vi "Read GUI Events.vi"(8 "error in (no error)":errorcluster, 11 "CS++Scope in":refnum<class "CS++Scope.lvclass">) -> (0 "error out":errorcluster, 2 "GUI Events":cluster{"Stop":refnum<user-event>}, 3 "CS++Scope out":refnum<class "CS++Scope.lvclass">)   [LabVIEW 2016, in "CS++Scope.lvlib" / "CS++Scope.lvclass"]
uses:
  CS++Scope.lvclass
  CS++Scope.lvclass/CS++Scope.ctl
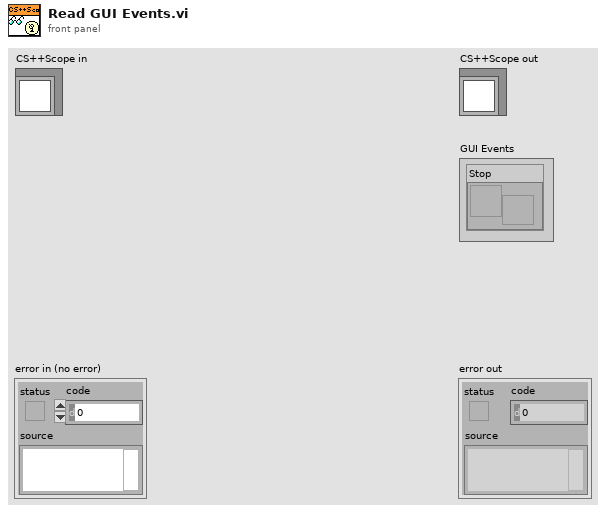
[diagram p1: front panel]
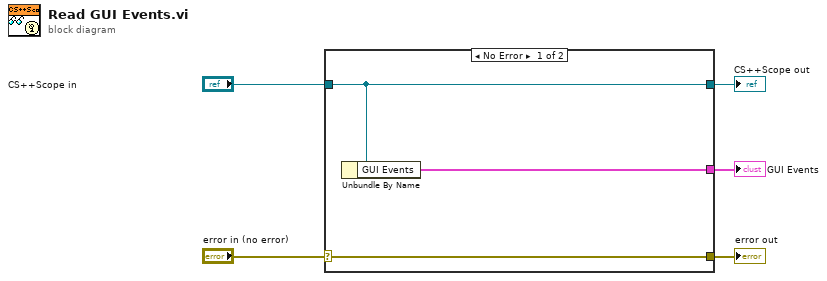
[diagram p0: block diagram]
diagram:
  n1 = case shown="No Error" "error in (no error)" {
    selector: "error in (no error)" -> [w8 w9]
    tunnel: [w8 w9] -> w4
    tunnel: [w7 w10] -> w2
    tunnel: "CS++Scope in" -> [w7 w10]
    tunnel: [w6 _] -> w1
    frame No Error {
      n2 = Unbundle By Name(w7) -> ("GUI Events"=w6:cluster{"Stop":refnum<user-event>})
    }
    frame Error {
    }
  }
  "error out" <- w4
  "CS++Scope out" <- w2
  "GUI Events" <- w1
